vi "SIMPID(v.2).vi"(3 "Range":dbl=10.0, 5 "upper limit":dbl=1.0, 7 "lower limit":dbl=0.4, 9 "Current Point":dbl(knob) scale=0.0..200.0, 10 "Set Point":dbl(knob) scale=0.0..200.0) -> (0 "On Target":bool, 1 "result":dbl)   [LabVIEW 2012]
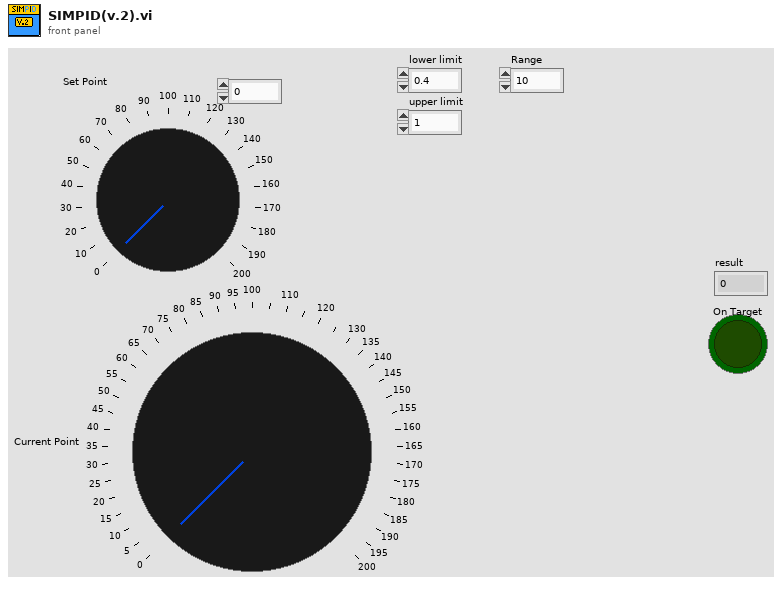
[diagram p1: front panel]
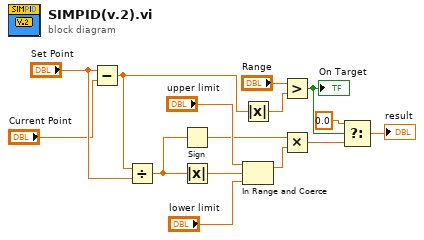
[diagram p0: block diagram]
diagram:
  n1 = Subtract(x="Set Point", y="Current Point") -> (x-y=w6:dbl)
  n2 = Divide(x=w6, y="Set Point") -> (x/y=w14:dbl)
  n3 = Sign(1:w14) -> (0:w12:dbl)
  n4 = Absolute Value(x=w14) -> (abs(x)=w15:dbl)
  n5 = Absolute Value(x=w6) -> (abs(x)=w11:dbl)
  n6 = In Range and Coerce(upper limit="upper limit", x=w15, lower limit="lower limit") -> (coerced(x)=w4:dbl)  [unwired: 1 out]
  n7 = Greater?(x="Range", y=w11) -> (0:w10:bool)
  "On Target" <- w10
  n8 = Multiply(x=w12, y=w4) -> (x*y=w7:dbl)
  n9 = Select(t=0.0, s=w10, f=w7) -> (s? t:f=→"result":dbl)
